vi "Query TrigSlope Core.vi"(8 "error in (no error)":errorcluster, 11 "CS++MCS in":refnum<class "CS++MCS.lvclass">) -> (0 "error out":errorcluster, 2 "TriggerSlope":u16, 3 "CS++MCS out":refnum<class "CS++MCS.lvclass">)   [LabVIEW 2016, in "CS++MCS.lvlib" / "CS++MCS.lvclass"]
doc: "This VI reads out the actual Trigger Slope from the device."
uses:
  CS++MCS.lvclass
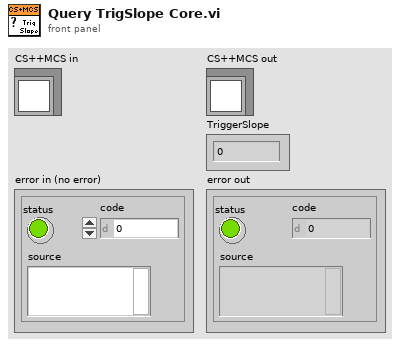
[diagram p1: front panel]
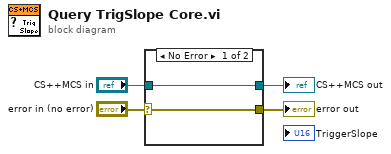
[diagram p0: block diagram]
diagram:
  n1 = case shown="No Error" "error in (no error)" {
    selector: "error in (no error)" -> [w6 w8]
    tunnel: [w6 w8] -> w3
    tunnel: [w5 w7] -> w1
    tunnel: "CS++MCS in" -> [w5 w7]
    frame No Error {
    }
    frame Error {
    }
  }
  "error out" <- w3
  "CS++MCS out" <- w1
